vi "Get Data Queue Ref.vi"(8 "error in (no error)":errorcluster) -> (0 "error out":errorcluster, 3 "Ground Station Operations Queue Ref":refnum<queue>)   [LabVIEW 2014]
uses:
  Controls/Data Queue.ctl
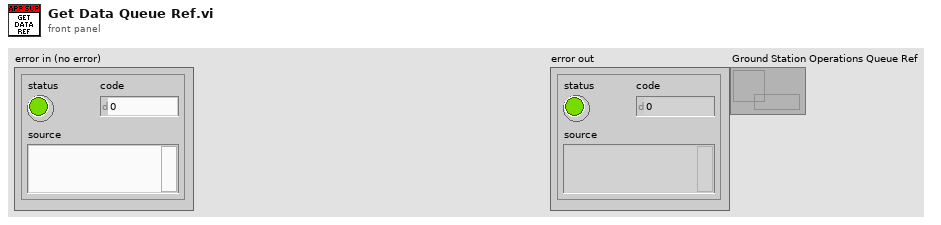
[diagram p1: front panel]
types:
  T1 = typedef "Data Queue.ctl" = cluster{"Command":string, "Data":variant}
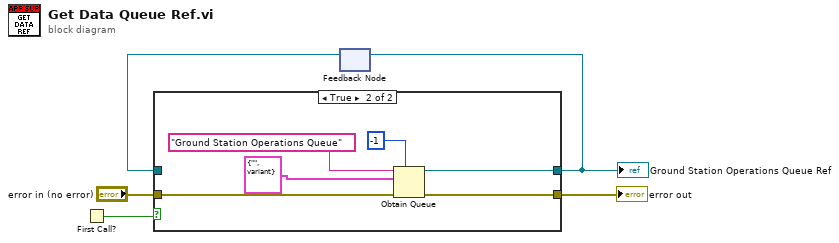
[diagram p0: block diagram]
diagram:
  n1 = First Call?() -> (First Call?: T/F=w4:bool)
  n2 = feedback #1() -> (w1:refnum<queue>)  [unwired: 1 in]
  n3 = case shown="True" w4 {
    tunnel: [w7 w12] -> w5
    tunnel: "error in (no error)" -> [w6 w11]
    tunnel: [w6 w10] -> w2
    tunnel: w1 -> [w7 _]
    frame False {
    }
    frame True {
      n4 = Obtain Queue(max queue size (-1, unlimited)=-1, name (unnamed)="Ground Station Operations Queue", element data type=T1 {"Command"="", "Data"=variant} ("Cluster"), error in (no error)=w11) -> (queue out=w12:refnum<queue>, error out=w10:errorcluster)  [unwired: 1 in, 1 out]
    }
  }
  "error out" <- w2
  "Ground Station Operations Queue Ref" <- w5
  n5 = feedback-in #1(w5) -> ()
